vi "AudioTest.Config, Get SoundCheck Data Plot Name Lookup.vi"(11 "Config Folder":path=path "C:/MTE/Audio Test/Config") -> (0 "error out":errorcluster, 3 "PlotNames":variant)   [LabVIEW 2018]
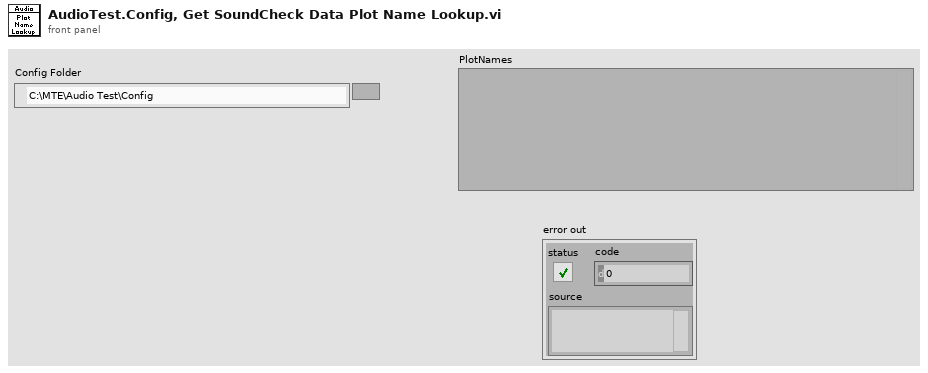
[diagram p1: front panel]
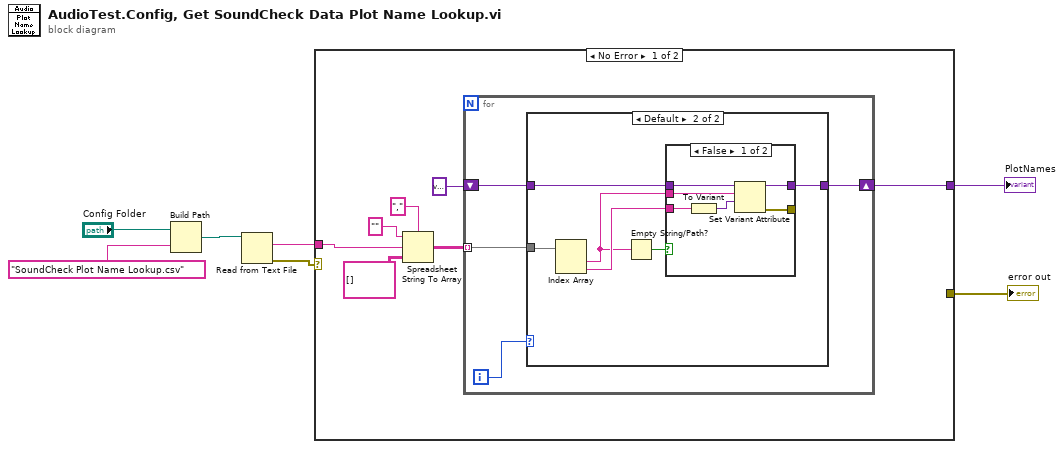
[diagram p0: block diagram]
diagram:
  n1 = Build Path(base path="Config Folder", name or relative path="SoundCheck Plot Name Lookup.csv") -> (appended path=w5:path)
  n2 = Read from Text File(file (use dialog)=w5) -> (text=w4:string, error out=w2:errorcluster)  [unwired: 3 in, 2 out]
  n3 = case shown="No Error" w2 {
    selector: w2 -> [_ w33]
    tunnel: w4 -> [w14 _]
    tunnel: [w8 _] -> w3
    tunnel: [_ w33] -> w1
    frame No Error {
      n4 = Spreadsheet String To Array(delimiter (Tab)=",", format string="", spreadsheet string=w14, array type (2D Dbl)=string[][] []) -> (array=w10:string[][])
      n5 = for {
        tunnel: w10 -> [w15] mode=indexing
        shift-right: [w16] -> w8
        shift-left: variant -> [w17]
        i -> [w18]
        n6 = case shown="Default" w18 {
          tunnel: w17 -> [w19 w25]
          tunnel: [w19 w24] -> w16
          tunnel: w15 -> [_ w23]
          frame 0 {
            # "Skip Heading"
          }
          frame Default {
            n7 = Index Array(array=w23) -> (element #1=w21:string, element #2=w22:string)  [unwired: 2 in]
            n8 = Empty String/Path?(string/path=w21) -> (empty?=w20:bool)
            n9 = case shown="False" w20 {
              tunnel: w25 -> [w31 w32]
              tunnel: [w30 w32] -> w24
              tunnel: w21 -> [w29 _]
              tunnel: w22 -> [w27 _]
              tunnel: [w26 _] -> _
              frame False {
                n10 = To Variant(anything=w27) -> (Variant=w28:variant)
                n11 = Set Variant Attribute(Variant=w31, name=w29, value=w28) -> (Variant out=w30:variant, error out=w26:errorcluster)  [unwired: 1 in, 1 out]
              }
              frame True {
              }
            }
          }
        }
      }
    }
    frame Error {
    }
  }
  "PlotNames" <- w3
  "error out" <- w1
